vi "CalculateProgress.vi"(4 "Voltage Index":i32, 5 "RTD Index":i32, 6 "Relay Index":i32, 7 "temp index":i32, 8 "Relay Settings":i32, 9 "RTD Temps":dbl[](array[numeric])=[50.0, 60.0, 70.0, 80.0, 90.0, 100.0, 110.0], 10 "Voltages":dbl[](array[numeric])=[18.0, 24.0, 36.0], 11 "Soak Temps":dbl[](array[numeric])=[25.0, 35.0]) -> (0 "Percent of Total":u8, 1 "Percent at Given Temp":u8, 2 "Index":dbl, 3 "Total":dbl)   [LabVIEW 2013]
panel:
  out "Total at Given Temp":dbl
  out "Index at Given Temp":dbl
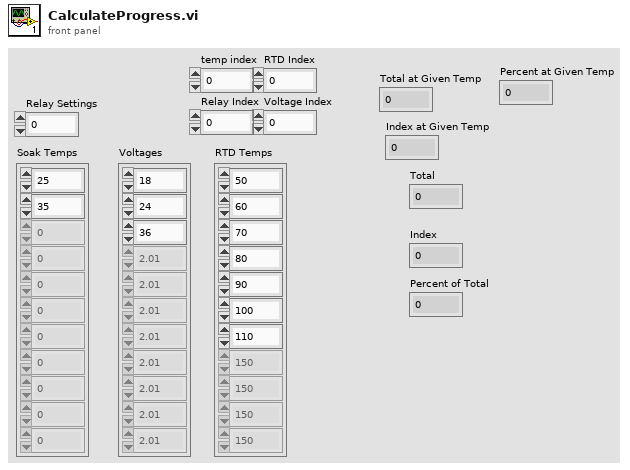
[diagram p1: front panel]
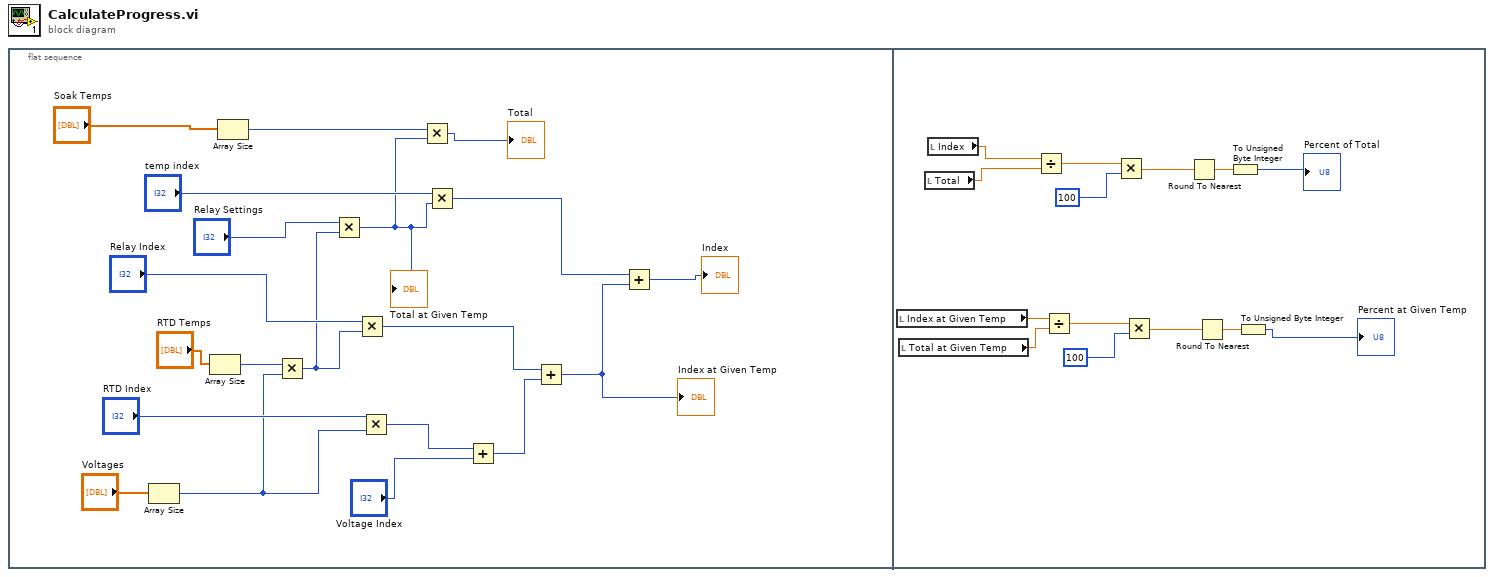
[diagram p0: block diagram]
diagram:
  n1 = flat-sequence {
    frame #0 {
      n2 = Array Size(array="Voltages") -> (size(s)=w7:i32)
      n3 = Array Size(array="RTD Temps") -> (size(s)=w8:i32)
      n4 = Array Size(array="Soak Temps") -> (size(s)=w9:i32)
      n5 = Multiply(x=w8, y=w7) -> (x*y=w14:i32)
      n6 = Multiply(x="Relay Settings", y=w14) -> (x*y=w2:i32)
      "Total at Given Temp" <- w2
      n7 = Multiply(x="Relay Index", y=w14) -> (x*y=w4:i32)
      n8 = Multiply(x="RTD Index", y=w7) -> (x*y=w18:i32)
      n9 = Multiply(x=w9, y=w2) -> (x*y=→"Total":i32)
      n10 = Multiply(x="temp index", y=w2) -> (x*y=w12:i32)
      n11 = Add(x=w18, y="Voltage Index") -> (x+y=w11:i32)
      n12 = Add(x=w4, y=w11) -> (x+y=w1:i32)
      "Index at Given Temp" <- w1
      n13 = Add(x=w12, y=w1) -> (x+y=→"Index":i32)
    }
    frame #1 {
      n14 = local read "Index at Given Temp"() -> (w32:dbl)
      n15 = local read "Total at Given Temp"() -> (w33:dbl)
      n16 = local read "Total"() -> (w30:dbl)
      n17 = local read "Index"() -> (w31:dbl)
      n18 = Divide(x=w31, y=w30) -> (x/y=w21:dbl)
      n19 = Divide(x=w32, y=w33) -> (x/y=w26:dbl)
      n20 = Multiply(x=w21, y=100) -> (x*y=w22:dbl)
      n21 = Multiply(x=w26, y=100) -> (x*y=w27:dbl)
      n22 = Round To Nearest(number=w22) -> (nearest integer value=w24:dbl)
      n23 = Round To Nearest(number=w27) -> (nearest integer value=w29:dbl)
      n24 = To Unsigned Byte Integer(number=w24) -> (unsigned 8bit integer=→"Percent of Total":u8)
      n25 = To Unsigned Byte Integer(number=w29) -> (unsigned 8bit integer=→"Percent at Given Temp":u8)
    }
  }
